vi "shift_rotate.vi"(5 "dy":dbl, 6 "dx":dbl, 7 "c_y":dbl, 8 "y":dbl, 9 "x":dbl, 10 "c_x":dbl, 11 "alpha":dbl) -> (2 "new_y":dbl, 3 "new_x":dbl)   [LabVIEW 2012]
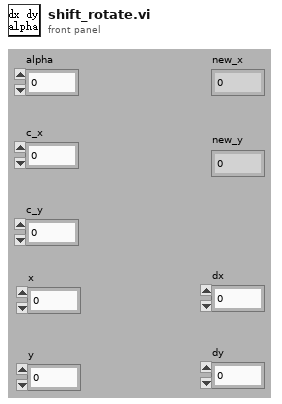
[diagram p1: front panel]
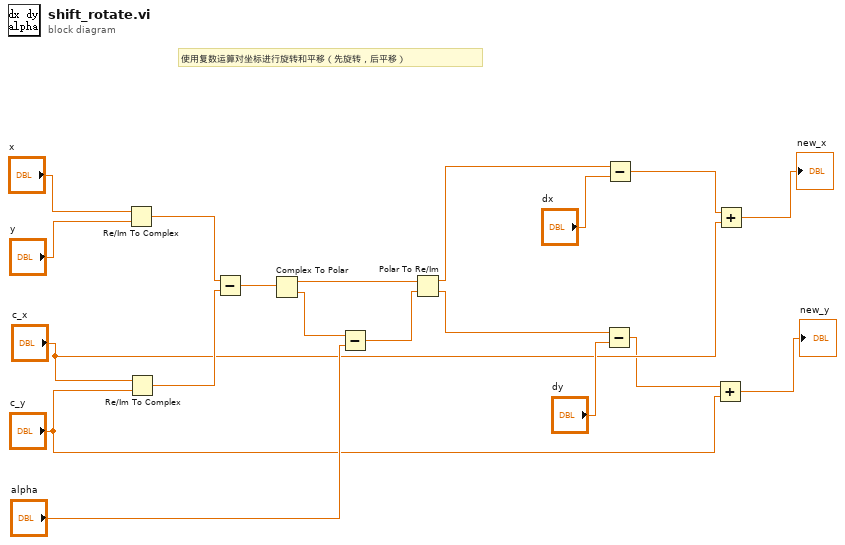
[diagram p0: block diagram]
diagram:
  # "使用复数运算对坐标进行旋转和平移（先旋转，后平移）"
  n1 = Re/Im To Complex(1:"y", 2:"x") -> (0:w17:cdb)
  n2 = Re/Im To Complex(1:"c_y", 2:"c_x") -> (0:w16:cdb)
  n3 = Subtract(x=w17, y=w16) -> (x-y=w15:cdb)
  n4 = Complex To Polar(r * e^(i*theta)=w15) -> (r=w12:dbl, theta=w14:dbl)
  n5 = Subtract(x=w14, y="alpha") -> (x-y=w11:dbl)
  n6 = Polar To Re/Im(2:w11, 3:w12) -> (0:w9:dbl, 1:w7:dbl)
  n7 = Subtract(x=w9, y="dy") -> (x-y=w2:dbl)
  n8 = Subtract(x=w7, y="dx") -> (x-y=w5:dbl)
  n9 = Add(x=w2, y="c_y") -> (x+y=→"new_y":dbl)
  n10 = Add(x=w5, y="c_x") -> (x+y=→"new_x":dbl)
